vi "Event Self.vi"(10 "Msg":refnum<class "Msg Strategy.lvclass">, 11 "Hello World Event in":refnum<class "Hello World Event.lvclass">) -> (3 "Hello World Event out":refnum<class "Hello World Event.lvclass">)   [LabVIEW 2021, in "Hello World Event.lvlib" / "Hello World Event.lvclass"]
uses:
  Hello World Event.lvclass
  jettl/Msg Strategy/Msg Strategy/Msg Strategy.lvclass
  Hello World Event.lvclass/Hello World Event.ctl
  jettl/jettl/Event Actor/Event Actor.lvclass
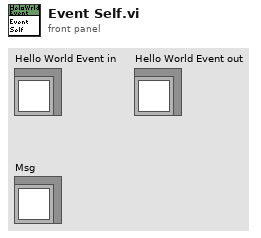
[diagram p1: front panel]
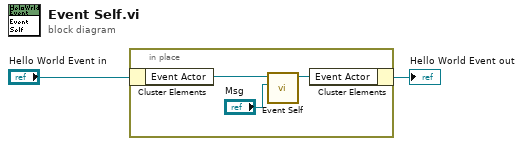
[diagram p0: block diagram]
diagram:
  n1 = in-place {
    n2 = in-place-cluster #1("Hello World Event in") -> ("Event Actor"=w5:refnum<class "Event Actor.lvclass">)
    n3 = call-dynamic "Event Self.vi"("Msg"="Msg", "Event Actor in"=w5) -> ("Event Actor out"=w4:refnum<class "Event Actor.lvclass">)  [unwired: 9 in]
    n4 = in-place-cluster #1("Event Actor"=w4) -> (→"Hello World Event out":refnum<class "Hello World Event.lvclass">)
  }
